vi "Write Key BOOL.vi"(7 "Section Name":string, 8 "error in":errorcluster, 9 "New Value":bool, 10 "Key Name":string, 11 "Config Cluster in":T1) -> (0 "error out":errorcluster, 3 "Config Cluster out":T1)   [LabVIEW 2017]
uses:
  Config Cluster.ctl
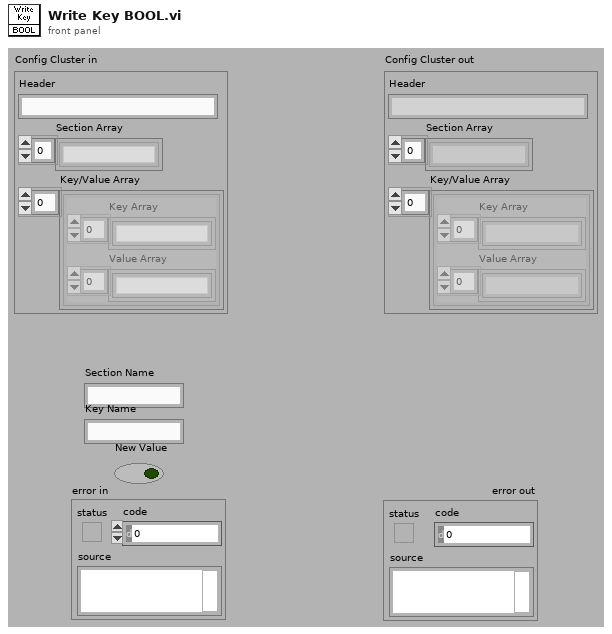
[diagram p1: front panel]
types:
  T1 = typedef "Config Cluster.ctl" = cluster{"Header":string, "Section Array":string[], "Key/Value Array":cluster{"Key Array":string[], "Value Array":string[]}[]}
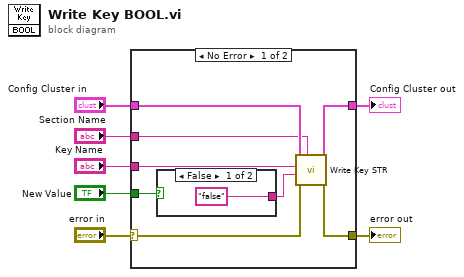
[diagram p0: block diagram]
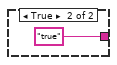
[diagram p2: hidden frame]
diagram:
  n1 = case shown="No Error" "error in" {
    selector: "error in" -> [w14 w18]
    tunnel: [w13 w18] -> w6
    tunnel: "Config Cluster in" -> [w11 w19]
    tunnel: [w12 w19] -> w4
    tunnel: "Section Name" -> [w10 _]
    tunnel: "Key Name" -> [w9 _]
    tunnel: "New Value" -> [w15 _]
    frame No Error {
      n2 = case shown="False" w15 {
        tunnel: ["false" "true"] -> w8
        frame False {
        }
        frame True {
        }
      }
      n3 = call "Write Key STR.vi"("Section Name"=w10, "error in"=w14, "New Value"=w8, "Key Name"=w9, "Config Cluster in"=w11) -> ("error out"=w13:errorcluster, "Config Cluster out"=w12:T1)  [unwired: 5 in]
    }
    frame Error {
    }
  }
  "error out" <- w6
  "Config Cluster out" <- w4
